vi "Write Gantry.vi"(8 "error in (no error)":errorcluster, 10 "Gantry Class.lvclass":refnum<class "Gantry Class.lvclass">, 11 "Tool Class in":refnum<class "Tool Class.lvclass">) -> (0 "error out":errorcluster, 3 "Tool Class out":refnum<class "Tool Class.lvclass">)   [LabVIEW 2011, in "Tool Class.lvclass"]
uses:
  Tool Class.lvclass
  Gantry Class/Gantry Class.lvclass
  Tool Class.lvclass/Tool Class.ctl
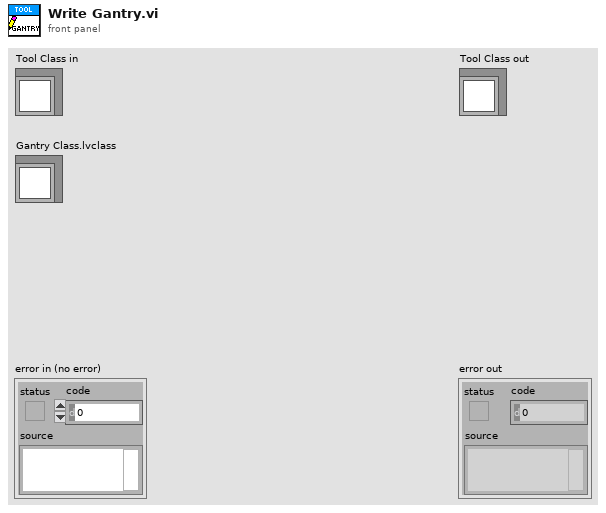
[diagram p1: front panel]
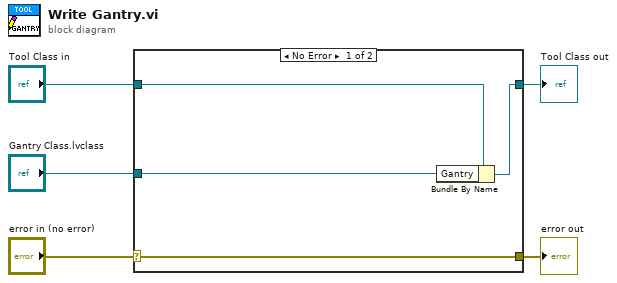
[diagram p0: block diagram]
diagram:
  n1 = case shown="No Error" "error in (no error)" {
    selector: "error in (no error)" -> [w9 w10]
    tunnel: [w9 w10] -> w4
    tunnel: [w7 w11] -> w2
    tunnel: "Tool Class in" -> [w8 w11]
    tunnel: "Gantry Class.lvclass" -> [w6 _]
    frame No Error {
      n2 = Bundle By Name(cluster=w8, "Gantry"=w6) -> (w7:refnum<class "Tool Class.lvclass">)
    }
    frame Error {
    }
  }
  "error out" <- w4
  "Tool Class out" <- w2
